vi "XYZStage-move command constructor.vi"(6 "Bypass Z-safety interlock":bool, 8 "error in (no error)":errorcluster, 9 "Z":sgl, 10 "Y":sgl, 11 "X":sgl) -> (0 "Move command":string, 1 "Adjusted Z":sgl, 2 "Adjusted Y":sgl, 3 "Adjusted X":sgl, 4 "error out":errorcluster)   [LabVIEW 2020]
uses:
  Typedefs/Z intelock check type.ctl
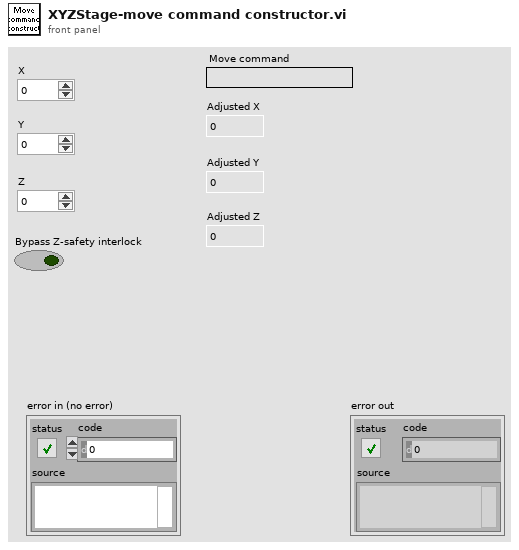
[diagram p1: front panel]
types:
  T1 = typedef "Z intelock check type.ctl" = enum16{"Check against Z limit", "Check againt current position"}
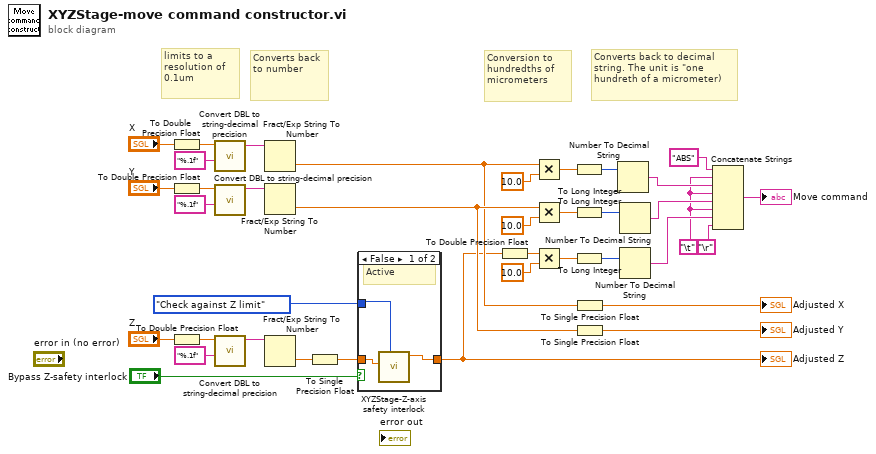
[diagram p0: block diagram]
diagram:
  w18 = "\t" ("Tab Constant")
  # "Converts back to decimal string. The unit is \"one hundreth of a micrometer)"
  # "Converts back to number"
  # "limits to a resolution of 0.1um"
  # "Conversion to hundredths of micrometers"
  n1 = To Double Precision Float(number="X") -> (double precision float=w5:dbl)
  n2 = To Double Precision Float(number="Y") -> (double precision float=w4:dbl)
  n3 = To Double Precision Float(number="Z") -> (double precision float=w3:dbl)
  n4 = call <userlib>:"Convert DBL to string-decimal precision.vi"("Format (%f)"="%.1f", "DBL Value"=w5) -> ("Converted to String"=w29:string)  [unwired: 9 in]
  n5 = call <userlib>:"Convert DBL to string-decimal precision.vi"("Format (%f)"="%.1f", "DBL Value"=w4) -> ("Converted to String"=w30:string)  [unwired: 9 in]
  n6 = call <userlib>:"Convert DBL to string-decimal precision.vi"("Format (%f)"="%.1f", "DBL Value"=w3) -> ("Converted to String"=w31:string)  [unwired: 9 in]
  n7 = Fract/Exp String To Number(string=w29) -> (number=w37:dbl)  [unwired: 3 in, 1 out]
  n8 = Fract/Exp String To Number(string=w30) -> (number=w38:dbl)  [unwired: 3 in, 1 out]
  n9 = Fract/Exp String To Number(string=w31) -> (number=w9:dbl)  [unwired: 3 in, 1 out]
  n10 = To Single Precision Float(number=w9) -> (single precision float=w7:sgl)
  n11 = case shown="False" "Bypass Z-safety interlock" {
    tunnel: [w41 w42] -> w8
    tunnel: w7 -> [w40 w42]
    tunnel: Z_intelock_check_type."Check against Z limit" ("Interlock check type") -> [w39 _]
    frame False {
      # "Active"
      n12 = call "XYZStage-Z-axis safety interlock.vi"("Interlock check type"=w39, "Z move to"=w40) -> ("Z"=w41:sgl)  [unwired: 8 in, 1 out]
    }
    frame True {
      # "Bypassed"
    }
  }
  "Adjusted Z" <- w8
  n13 = To Double Precision Float(number=w8) -> (double precision float=w6:dbl)
  n14 = Multiply(x=w37, y=10.0) -> (x*y=w13:dbl)
  n15 = Multiply(x=w38, y=10.0) -> (x*y=w33:dbl)
  n16 = Multiply(x=w6, y=10.0) -> (x*y=w35:dbl)
  n17 = To Long Integer(number=w13) -> (32bit integer=w12:i32)
  n18 = To Long Integer(number=w33) -> (32bit integer=w11:i32)
  n19 = To Long Integer(number=w35) -> (32bit integer=w10:i32)
  n20 = To Single Precision Float(number=w37) -> (single precision float=→"Adjusted X":sgl)
  n21 = To Single Precision Float(number=w38) -> (single precision float=→"Adjusted Y":sgl)
  n22 = Number To Decimal String(number=w12) -> (decimal integer string=w32:string)  [unwired: 1 in]
  n23 = Number To Decimal String(number=w11) -> (decimal integer string=w34:string)  [unwired: 1 in]
  n24 = Number To Decimal String(number=w10) -> (decimal integer string=w36:string)  [unwired: 1 in]
  n25 = Concatenate Strings("ABS" ("decimal integer string"), w18, w32, w18, w34, w18, w36, "\r" ("Carriage Return Constant")) -> (→"Move command":string)
